vi "PQfsize.vi"(7 "error in (no error)":errorcluster, 9 "field_num":u32, 10 "res":u32) -> (0 "error out":errorcluster, 2 "size":i32, 3 "res_out":u32)   [LabVIEW 2019, in "libpqlv.lvlib"]
doc: "Returns the size in bytes of the column associated with the given column number. Column numbers start at 0.\n\nPQfsize returns the space allocated for this column in a database row, in other words the size of the server's internal representation of the data type. (Accordingly, it is not really very useful to clients.) A negative value indicates the data type is variable-length."
uses:
  libpqlv.lvlib
  libpq.dll
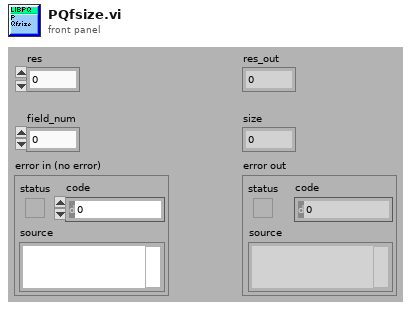
[diagram p1: front panel]
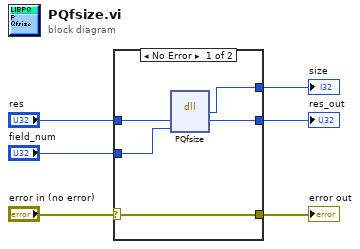
[diagram p0: block diagram]
diagram:
  n1 = case shown="No Error" "error in (no error)" {
    selector: "error in (no error)" -> [w11 w13]
    tunnel: [w11 w13] -> w5
    tunnel: [w10 _] -> w4
    tunnel: "field_num" -> [w9 _]
    tunnel: "res" -> [w8 w12]
    tunnel: [w7 w12] -> w1
    frame No Error {
      n2 = dll-call lib="libpq.*" fn="PQfsize"("res"=w8, "field_num"=w9) -> ("size"=w10:i32, "res"=w7:u32)  [unwired: 4 in, 2 out]
    }
    frame Error {
    }
  }
  "size" <- w4
  "error out" <- w5
  "res_out" <- w1
